vi "test_Task Actor1.vi"(8 "Error in":errorcluster) -> (0 "error out":errorcluster)   [LabVIEW 2023]
uses:
  Task Actor/Task Actor.lvclass
  Task Base/Task Base.lvclass
  Task Base/Task Base.lvclass/Task Base.ctl
  Task Actor/Task Actor.lvclass/Task Actor.ctl
  <vilib>/ActorFramework/Message Enqueuer/Message Enqueuer.lvclass/Message Enqueuer.ctl
  <vilib>/ActorFramework/Stop Msg/Stop Msg.lvclass/Stop Msg.ctl
  <vilib>/ActorFramework/Message Enqueuer/Enqueue.vi
  <vilib>/ActorFramework/Message Enqueuer/Enqueue Critical.vi
  ITask Actor/ITask Actor Messages/Perform Action Msg/Perform Action Msg.lvclass
  <vilib>/ActorFramework/Stop Msg/Stop Msg.lvclass
  <vilib>/Utility/error.llb/Error Cluster From Error Code.vi
  <vilib>/Utility/LVClass/Get LV Class Name.vi
  <resource>/AFDebug/Generate Trace for Message.vi
  <vilib>/ActorFramework/Message Priority Queue/Priority Enqueue.vi
  <vilib>/ActorFramework/Actor/Actor.lvclass
  Measure and Stimulus Subsystems/Measure and Stimulus Subsystems.lvclass
panel:
  in  "Shutdown Actor":bool
  out "WF Chart":waveform(dbl)(graph)
  out "WF Chart Lossy":waveform(dbl)(graph)
  in  "Stop":bool
  in  "Perform Action":bool
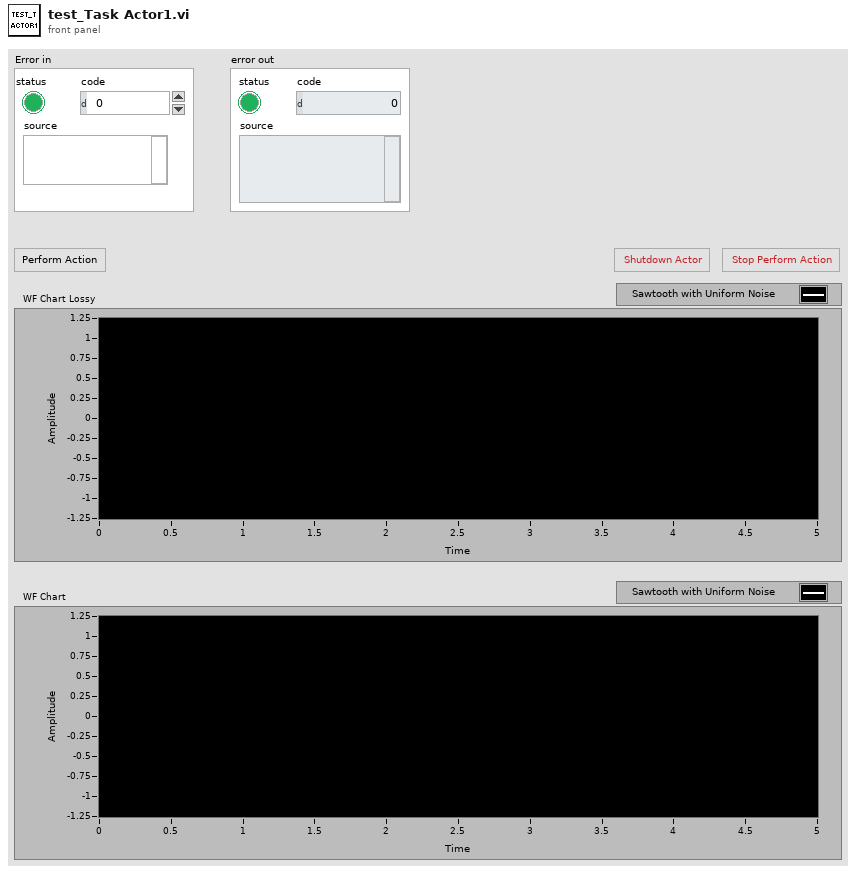
[diagram p1: front panel]
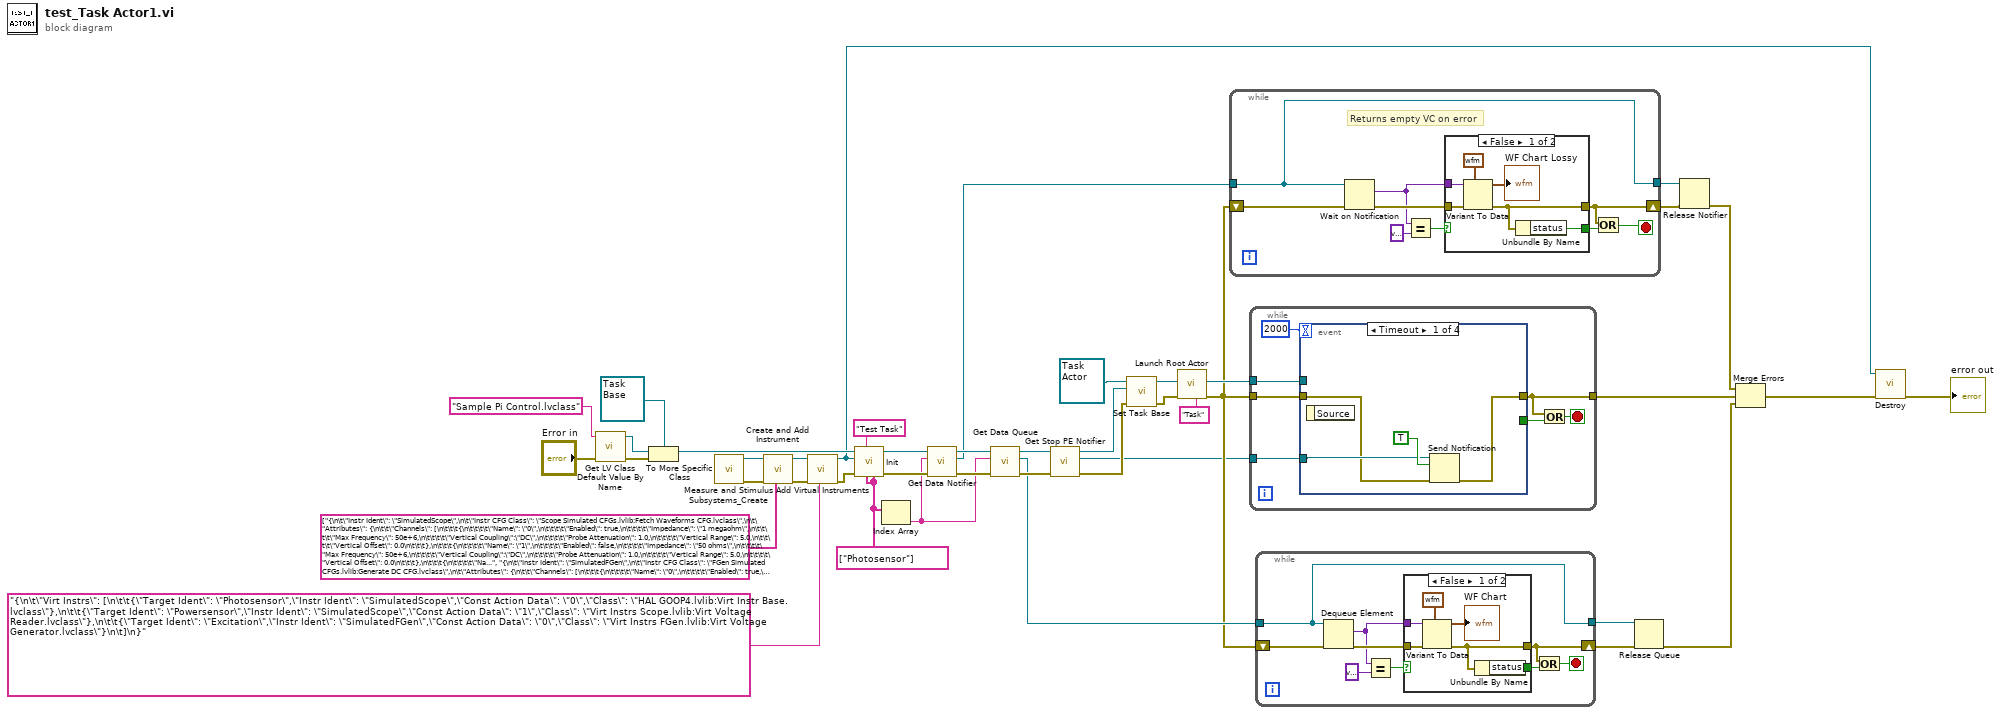
[diagram p0: block diagram]
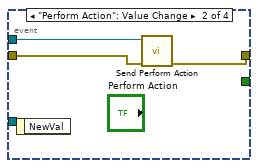
[diagram p4: hidden frame]
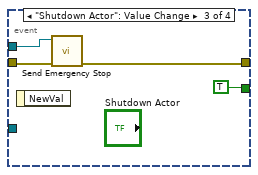
[diagram p5: hidden frame]
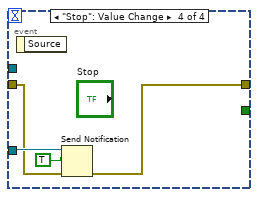
[diagram p6: hidden frame]
diagram:
  w10 = string[] ["Photosensor"] ("Data Notifier Names")
  n1 = call <vilib>:"Get LV Class Default Value By Name.vi"("error in (no error)"="Error in", "class name"="Sample Pi Control.lvclass") -> ("error out"=w38:errorcluster, "object"=w39:refnum<class>)  [unwired: 8 in]
  n2 = To More Specific Class(target class=refnum<class "Task Base.lvclass"> refnum ("HAL GOOP4.lvlib:Task Base.lvclass"), reference=w39, error in=w38) -> (specific class reference=w36:refnum<class "Task Base.lvclass">)  [unwired: 1 out]
  n3 = call "Measure and Stimulus Subsystems_Create.vi"() -> ("Error Out"=w35:errorcluster, "reference out"=w6:refnum<class "Measure and Stimulus Subsystems.lvclass">)  [unwired: 10 in]
  n4 = call "Create and Add Instrument.vi"("Physical Intr Configs"=string[] ["{\n\t\"Instr Ident\": \"SimulatedScope\",\n\t\"Instr CFG Class\": \"Scope Simulated CFGs.lvlib:Fetch Waveforms CFG.lvclass\",\n\t\"Attributes\": {\n\t\t\"Channels\": [\n\t\t\t{\n\t\t\t\t\"Name\": \"0\",\n\t\t\t\t\"Enabled\": true,\n\t\t\t\t\"Impedance\": \"1 megaohm\",\n\t\t\t\t\"Max Frequency\": 50e+6,\n\t\t\t\t\"Vertical Coupling\":\"DC\",\n\t\t\t\t\"Probe Attenuation\": 1.0,\n\t\t\t\t\"Vertical Range\": 5.0,\n\t\t\t\t\"Vertical Offset\": 0.0\n\t\t\t},\n\t\t\t{\n\t\t\t\t\"Name\": \"1\",\n\t\t\t\t\"Enabled\": false,\n\t\t\t\t\"Impedance\": \"50 ohms\",\n\t\t\t\t\"Max Frequency\": 50e+6,\n\t\t\t\t\"Vertical Coupling\":\"DC\",\n\t\t\t\t\"Probe Attenuation\": 1.0,\n\t\t\t\t\"Vertical Range\": 5.0,\n\t\t\t\t\"Vertical Offset\": 0.0\n\t\t\t},\n\t\t\t{\n\t\t\t\t\"Name\": \"2\",\n\t\t\t\t\"Enabled\": false,\n\t\t\t\t\"Impedance\": \"50 ohms\",\n\t\t\t\t\"Max Frequency\": 50e+6,\n\t\t\t\t\"Vertical Coupling\":\"DC\",\n\t\t\t\t\"Probe Attenuation\": 1.0,\n\t\t\t\t\"Vertical Range\": 5.0,\n\t\t\t\t\"Vertical Offset\": 0.0\n\t\t\t},\n\t\t\t{\n\t\t\t\t\"Name\": \"3\",\n\t\t\t\t\"Enabled\": true,\n\t\t\t\t\"Impedance\": \"50 ohms\",\n\t\t\t\t\"Max Frequency\": 50e+6,\n\t\t\t\t\"Vertical Coupling\":\"DC\",\n\t\t\t\t\"Probe Attenuation\": 1.0,\n\t\t\t\t\"Vertical Range\": 1.4,\n\t\t\t\t\"Vertical Offset\": 0.0\n\t\t\t},\n\t\t\t{\n\t\t\t\t\"Name\": \"4\",\n\t\t\t\t\"Enabled\": false,\n\t\t\t\t\"Impedance\": \"50 ohms\",\n\t\t\t\t\"Max Frequency\": 50e+6,\n\t\t\t\t\"Vertical Coupling\":\"DC\",\n\t\t\t\t\"Probe Attenuation\": 1.0,\n\t\t\t\t\"Vertical Range\": 5.0,\n\t\t\t\t\"Vertical Offset\": 0.0\n\t\t\t},\n\t\t\t{\n\t\t\t\t\"Name\": \"5\",\n\t\t\t\t\"Enabled\": false,\n\t\t\t\t\"Impedance\": \"50 ohms\",\n\t\t\t\t\"Max Frequency\": 50e+6,\n\t\t\t\t\"Vertical Coupling\":\"DC\",\n\t\t\t\t\"Probe Attenuation\": 1.0,\n\t\t\t\t\"Vertical Range\": 5.0,\n\t\t\t\t\"Vertical Offset\": 0.0\n\t\t\t},\n\t\t\t{\n\t\t\t\t\"Name\": \"6\",\n\t\t\t\t\"Enabled\": false,\n\t\t\t\t\"Impedance\": \"50 ohms\",\n\t\t\t\t\"Max Frequency\": 50e+6,\n\t\t\t\t\"Vertical Coupling\":\"DC\",\n\t\t\t\t\"Probe Attenuation\": 1.0,\n\t\t\t\t\"Vertical Range\": 5.0,\n\t\t\t\t\"Vertical Offset\": 0.0\n\t\t\t},\n\t\t\t{\n\t\t\t\t\"Name\": \"7\",\n\t\t\t\t\"Enabled\": false,\n\t\t\t\t\"Impedance\": \"50 ohms\",\n\t\t\t\t\"Max Frequency\": 50e+6,\n\t\t\t\t\"Vertical Coupling\":\"DC\",\n\t\t\t\t\"Probe Attenuation\": 1.0,\n\t\t\t\t\"Vertical Range\": 5.0,\n\t\t\t\t\"Vertical Offset\": 0.0\n\t\t\t}\n\t\t],\n\t\t\"Horizontal\": {\n\t\t\t\"Enforce Realtime\": true,\n\t\t\t\"Number of Records\": 1,\n\t\t\t\"Min Sample Rate\": 1e+5,\n\t\t\t\"Reference Position\":50, //percent\n\t\t\t\"Min Record Length\":1e+3\n\t\t},\n\t\t\"Acquire\": {\n\t\t\t\"Type\": \"Normal\",\n\t\t\t\"NumSamples\": 1e+3,\n\t\t\t\"Fetch Relative To\": \"Read Pointer\"\n\t\t},\n\t\t\"Export Signal\": {\n\t\t\t\"Signal Identifier\": \"None\",\n\t\t\t\"Signal\": \"None\",\n\t\t\t\"Output Terminal\": \"None\"\n\t\t},\n\t\t\"Trigger\": {\n\t\t\t\"Type\": \"Immediate\",\n\t\t\t\"Slope\": \"Positive\",\n\t\t\t\"Source\": \"RTSI 0\",\n\t\t\t\"Holdoff\": 0.0,\n\t\t\t\"Delay\": 0.0\n\t\t}\n\t}\n}", "{\n\t\"Instr Ident\": \"SimulatedFGen\",\n\t\"Instr CFG Class\": \"FGen Simulated CFGs.lvlib:Generate DC CFG.lvclass\",\n\t\"Attributes\": {\n\t\t\"Channels\": [\n\t\t\t{\n\t\t\t\t\"Name\": \"0\",\n\t\t\t\t\"Enabled\": true,\n\t\t\t\t\"Waveform\": \"DC\",\n\t\t\t\t\"Frequency\": 0, //DC\n\t\t\t\t\"Amplitude\": 0.0,\n\t\t\t\t\"Start Phase\": 0.0,\n\t\t\t\t\"DC Offset\": 0.0,\n\t\t\t\t\"Trigger Mode\": \"Single\"\n\t\t\t}\n\t\t],\n\t\t\"Export Signal\": {\n\t\t\t\"Enabled\": true,\n\t\t\t\"Output Terminal\": \"PFI 0\",\n\t\t\t\"Signal Identifier\": \"None\",\n\t\t\t\"Signal\": \"Start Trigger\"\n\t\t}\n\t}\n}"], "Error In"=w35, "reference in"=w6) -> ("Error Out"=w34:errorcluster, "reference out"=w30:refnum<class "Measure and Stimulus Subsystems.lvclass">)  [unwired: 7 in]
  n5 = call "Add Virtual Instruments.vi"("<JSON CFG>"="{\n\t\"Virt Instrs\": [\n\t\t{\"Target Ident\": \"Photosensor\",\"Instr Ident\": \"SimulatedScope\",\"Const Action Data\": \"0\",\"Class\": \"HAL GOOP4.lvlib:Virt Instr Base.lvclass\"},\n\t\t{\"Target Ident\": \"Powersensor\",\"Instr Ident\": \"SimulatedScope\",\"Const Action Data\": \"1\",\"Class\": \"Virt Instrs Scope.lvlib:Virt Voltage Reader.lvclass\"},\n\t\t{\"Target Ident\": \"Excitation\",\"Instr Ident\": \"SimulatedFGen\",\"Const Action Data\": \"0\",\"Class\": \"Virt Instrs FGen.lvlib:Virt Voltage Generator.lvclass\"}\n\t]\n}", "Error In"=w34, "reference in"=w30) -> ("Error Out"=w33:errorcluster, "reference out"=w5:refnum<class "Measure and Stimulus Subsystems.lvclass">)  [unwired: 7 in]
  n6 = call-dynamic "Init.vi"("Data Queue Names"=w10, "Data Notifier Names"=w10, "Name"="Test Task", "error in (no error)"=w33, "MSS"=w5, "Task Base in"=w36) -> ("error out"=w29:errorcluster, "Task Base out"=w17:refnum<class "Task Base.lvclass">)  [unwired: 4 in]
  n7 = Index Array(array=w10) -> (element=w9:string)  [unwired: 1 in]
  n8 = call "Get Data Notifier.vi"("error in (no error)"=w29, "Target Name"=w9, "Task Base in"=w17) -> ("error out"=w18:errorcluster, "Data Notifier"=w12:refnum<notifier>, "Task Base out"=w15:refnum<class "Task Base.lvclass">)  [unwired: 6 in]
  n9 = call "Get Data Queue.vi"("error in (no error)"=w18, "Target Name"=w9, "Task Base in"=w15) -> ("error out"=w16:errorcluster, "Data Queue"=w14:refnum<queue>, "Task Base out"=w3:refnum<class "Task Base.lvclass">)  [unwired: 6 in]
  n10 = call "Get Stop PE Notifier.vi"("error in (no error)"=w16, "Task Base in"=w3) -> ("error out"=w4:errorcluster, "Stop PE"=w1:refnum<notifier>, "Task Base out"=w2:refnum<class "Task Base.lvclass">)  [unwired: 7 in]
  n11 = call "Set Task Base.vi"("error in (no error)"=w4, "HAL GOOP4.lvlib:Task Base.lvclass"=w2, "Task Actor in"=refnum<class "Task Actor.lvclass"> refnum ("Task Actor.lvlib:Task Actor.lvclass")) -> ("error out"=w28:errorcluster, "Task Actor out"=w42:refnum<class "Task Actor.lvclass">)  [unwired: 7 in]
  n12 = call <vilib>:"Launch Root Actor.vi"("Debug Alias"="Task", "error in (no error)"=w28, "Actor"=w42) -> ("error out"=w13:errorcluster, "Actor's Enqueuer"=w27:refnum<class "Message Enqueuer.lvclass">)  [unwired: 7 in]
  n13 = while {
    tunnel: w12 -> [w44]
    shift-right: [w48] -> w24
    shift-left: w13 -> [w50]
    tunnel: [w44] -> w8
    stop <- w49 stop-if-true
    # "Returns empty VC on error"
    n14 = Wait on Notification(notifier=w44, error in (no error)=w50) -> (notification=w51:variant, error out=w52:errorcluster)  [unwired: 2 in, 2 out]
    n15 = Equal?(x=w51, y=variant) -> (x = y?=w46:bool)
    n16 = case shown="False" w46 {
      selector: w46 -> [_ w60]
      tunnel: w52 -> [w58 w59]
      tunnel: [w54 w59] -> w48
      tunnel: w51 -> [w55 _]
      tunnel: [w53 w60] -> w45
      frame False {
        n17 = Variant To Data(error in=w58, type=waveform(dbl) {"t0"=timestamp(0 s since 1904-01-01), "dt"=1.0, "Y"=[]} ("Waveform"), Variant=w55) -> (data=→"WF Chart Lossy":waveform(dbl), error out=w54:errorcluster)
        n18 = Unbundle By Name(w54) -> ("status"=w53:bool)
      }
      frame True {
      }
    }
    n19 = Or(x=w48, y=w45) -> (x .or. y?=w49:bool)
  }
  n20 = while {
    tunnel: w27 -> [w67]
    tunnel: w13 -> [w66]
    tunnel: [w65] -> w25
    tunnel: w1 -> [w62]
    stop <- w64 stop-if-true
    n21 = event shown="[0] Timeout" {
      selector: _ -> [_ _ _ _]
      dyn-events: _ -> [_ _ _ _]
      timeout: 2000 -> [_ _ _ _]
      tunnel: w67 -> [_ w74 w77 _]
      tunnel: w66 -> [w69 w73 w78 w81]
      tunnel: [w68 w72 w76 w79] -> w65
      tunnel: [_ _ TRUE _] -> w63
      tunnel: w62 -> [w70 _ _ w82]
      event Timeout {
        n22 = event-data() -> ()  [unwired: 1 in, 1 out]
        n23 = Send Notification(notification=TRUE, notifier=w70, error in (no error)=w69) -> (error out=w68:errorcluster)  [unwired: 1 out]
      }
      event "Perform Action": Value Change {
        n24 = event-data() -> ()  [unwired: 1 in, 1 out]
        n25 = call "Send Perform Action.vi"("error in (no error)"=w73, "Message Enqueuer"=w74) -> ("error out"=w72:errorcluster)  [unwired: 8 in, 1 out]
      }
      event "Shutdown Actor": Value Change {
        n26 = event-data() -> ()  [unwired: 1 in, 1 out]
        n27 = call <vilib>:"Send Emergency Stop.vi"("error in (no error)"=w78, "Message Enqueuer"=w77) -> ("error out"=w76:errorcluster)  [unwired: 9 in]
      }
      event "Stop": Value Change {
        n28 = event-data() -> ()  [unwired: 1 in, 1 out]
        n29 = Send Notification(notification=TRUE, notifier=w82, error in (no error)=w81) -> (error out=w79:errorcluster)  [unwired: 1 out]
      }
    }
    n30 = Or(x=w65, y=w63) -> (x .or. y?=w64:bool)
  }
  n31 = while {
    tunnel: w14 -> [w86]
    tunnel: [w86] -> w20
    shift-right: [w83] -> w21
    shift-left: w13 -> [w85]
    stop <- w84 stop-if-true
    n32 = Dequeue Element(queue=w86, error in (no error)=w85) -> (element=w90:variant, error out=w91:errorcluster)  [unwired: 1 in, 2 out]
    n33 = Equal?(x=w90, y=variant) -> (x = y?=w88:bool)
    n34 = case shown="False" w88 {
      selector: w88 -> [_ w99]
      tunnel: w91 -> [w97 w98]
      tunnel: [w93 w98] -> w83
      tunnel: w90 -> [w94 _]
      tunnel: [w92 w99] -> w87
      frame False {
        n35 = Variant To Data(error in=w97, type=waveform(dbl) {"t0"=timestamp(0 s since 1904-01-01), "dt"=1.0, "Y"=[]} ("Waveform"), Variant=w94) -> (data=→"WF Chart":waveform(dbl), error out=w93:errorcluster)
        n36 = Unbundle By Name(w93) -> ("status"=w92:bool)
      }
      frame True {
      }
    }
    n37 = Or(x=w83, y=w87) -> (x .or. y?=w84:bool)
  }
  n38 = Release Queue(queue=w20, error in (no error)=w21) -> (error out=w19:errorcluster)  [unwired: 1 in, 2 out]
  n39 = Release Notifier(notifier=w8, error in (no error)=w24) -> (error out=w23:errorcluster)  [unwired: 1 in, 2 out]
  n40 = Merge Errors(w23, w25, w19) -> (w22:errorcluster)
  n41 = call "Destroy.vi"("Error In"=w22, "reference in"=w5) -> ("Error Out"=→"error out":errorcluster)  [unwired: 8 in, 1 out]
